vi "test data changed vi.vi"() -> ()   [LabVIEW 2017]
uses:
  36fe06a0-c2ca-47c7-af80-d05a4a7253ae.vi
  e94423ed-0b32-47c0-ac5f-a57f4f6257db.vi
  16e37ef2-3af0-403d-816a-be1640b23fe2.vi
  ce162119-3d4b-4443-9623-e0c9b2fa43ea.vi
panel:
  in  "go":bool
  out "str first call ignore":bool
  out "str first call included":bool
  out "array first call ignore":bool
  out "array first call included":bool
  in  "Array":string[](array[string])
  in  "String":string
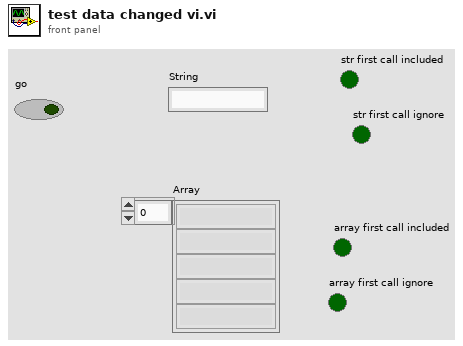
[diagram p1: front panel]
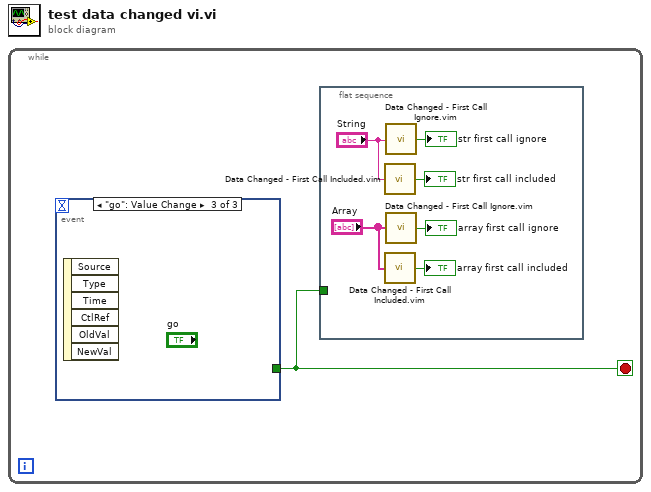
[diagram p0: block diagram]
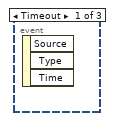
[diagram p2: hidden frame]
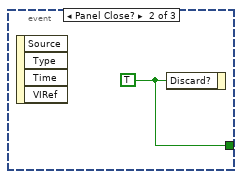
[diagram p3: hidden frame]
diagram:
  n1 = while {
    stop <- w1 stop-if-true
    n2 = event shown="[2] \"go\": Value Change" {
      selector: _ -> [_ _ _]
      dyn-events: _ -> [_ _ _]
      timeout: _ -> [_ _ _]
      tunnel: [_ w8 _] -> w1
      event Timeout {
        n3 = event-data() -> ()  [unwired: 1 in, 3 out]
      }
      event Panel Close? {
        w8 = TRUE ("Discard?")
        n4 = event-data() -> ()  [unwired: 1 in, 4 out]
        n5 = event-data("Discard?"=w8) -> ()  [unwired: 1 in, 1 out]
      }
      event "go": Value Change {
        n6 = event-data() -> ()  [unwired: 1 in, 6 out]
      }
    }
    n7 = flat-sequence {
      tunnel: w1 -> [_]
      frame #0 {
        n8 = call "Data Changed - First Call Included.vim"("Variant"="String") -> ("Changed"=→"str first call included":bool)
        n9 = call "Data Changed - First Call Included.vim"("Variant"="Array") -> ("Changed"=→"array first call included":bool)
        n10 = call "Data Changed - First Call Ignore.vim"("Variant"="String") -> ("Changed"=→"str first call ignore":bool)
        n11 = call "Data Changed - First Call Ignore.vim"("Variant"="Array") -> ("Changed"=→"array first call ignore":bool)
      }
    }
  }
